vi "User_Database_SQL.vi"(7 "Get Record":bool=TRUE, 8 "error in (no error)":errorcluster caption="错误输入（无错误）", 10 "SQL query":string) -> (0 "error out":errorcluster caption="错误输出", 1 "Null?":bool, 2 "Record":string[][](array[string]))   [LabVIEW 2020]
panel:
  in  "db Path":path=path "G:/2023项目/陆译电子/0008 User Management/Config/User_Info/User_Info.db"
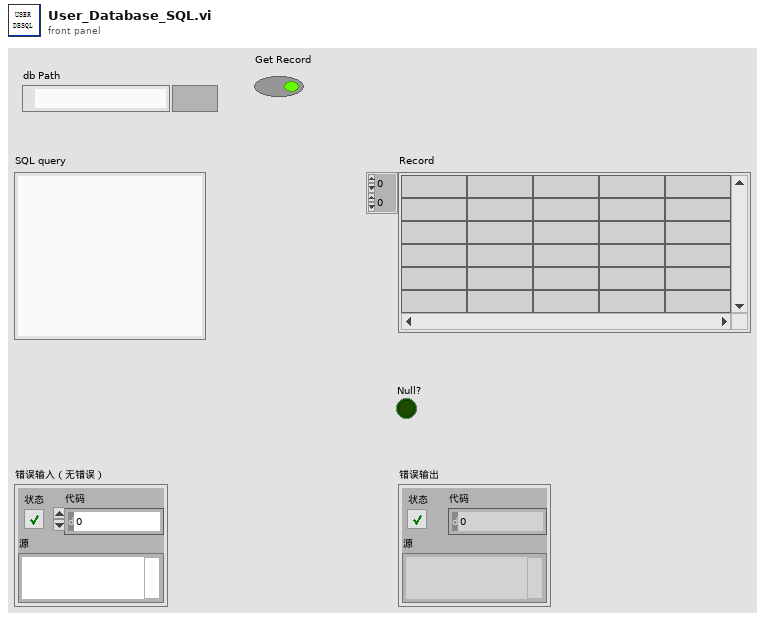
[diagram p1: front panel]
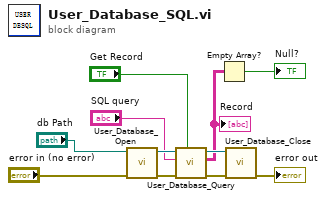
[diagram p0: block diagram]
diagram:
  n1 = call "User_Database_Open.vi"("error in (no error)"="error in (no error)", "db Path"="db Path") -> ("error out"=w7:errorcluster, "SQLite Connection"=w8:refnum<class "Connection.lvclass">)  [unwired: 8 in]
  n2 = call "User_Database_Query.vi"("Read?"="Get Record", "error in (no error)"=w7, "SQL query"="SQL query", "SQLite Connection in"=w8) -> ("error out"=w3:errorcluster, "Data"=w2:string[][], "SQLite Connection"=w4:refnum<class "Connection.lvclass">)  [unwired: 5 in]
  "Record" <- w2
  n3 = Empty Array?(array=w2) -> (empty?=→"Null?":bool)
  n4 = call "User_Database_Close.vi"("error in (no error)"=w3, "SQLite Connection in"=w4) -> ("error out"=→"error out":errorcluster)  [unwired: 9 in]
